vi "mult.vi"(1 "y":i16, 2 "x":i16) -> (0 "x*y":i32)   [LabVIEW 2017]
doc: "Multiplies two 16-bit numbers to yield a 32-bit result without integer overflow by returning a maximum or minimum value."
uses:
  <vilib>/rvi/Arithmetic/AddSubMult/XNode/nirviSatArithmetic.xnode
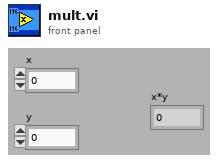
[diagram p1: front panel]
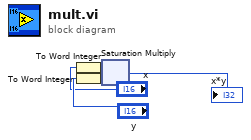
[diagram p0: block diagram]
diagram:
  n1 = To Word Integer(number="x") -> (16bit integer=w1:i16)
  n2 = To Word Integer(number="y") -> (16bit integer=w2:i16)
  n3 = xnode "Saturation Multiply"("x"=w1, "y"=w2) -> ("x*y"=→"x*y":i32)
